vi "Thorlabs_TDC001.findReference.vi"(0 "i ref in":refnum<vi>, 5 "error in (no error)":errorcluster) -> (14 "i ref out":refnum<vi>, 19 "error out":errorcluster)   [LabVIEW 2014, in "Thorlabs_TDC001.lvlib"]
doc: "This is the constructor of a class.\n\nLicense Agreement for this software:\n\nCopyright (C)\nGesellschaft für Schwerionenforschung, GSI\nPlanckstr. 1\n64291 Darmstadt\nGermany\n\nContact: D.Beck@gsi.de \n\nThis program is free software; you can redistribute it and/or modify it under the terms of the \nGNU General Public License as published by the Free Software Foundation; either version 2 of \nthe license, or (at your option) any later version.\n\nThis program is distributed in the hope that it will be useful, but WITHOUT ANY WARRANTY; \nwithout even the implied warranty of MERCHANTABILITY or FITNESS FOR A PARTICULAR PURPOSE. See the GNU General License for more details (http://www.gnu.org).\n\nGesellschaft für Schwerionenforschung, GSI\nPlanckstr. 1, 64291 Darmstadt, Germany\nFor all questions and ideas contact: M.Richter@gsi.de, H.Brand@gsi.de or D.Beck@gsi.de.\nLast update: 16-JUN-2004"
uses:
  Thorlabs_TDC001.lvlib
panel:
  in  "MG17Motor":refnum<k7>(container)
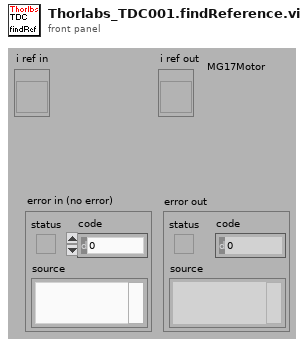
[diagram p1: front panel]
types:
  T1 = typedef "Thorlabs_TDC001.lvlib/Thorlabs_TDC001.i attribute.ctl" = cluster{"SerialNo":i32, "ChannelID":i32}
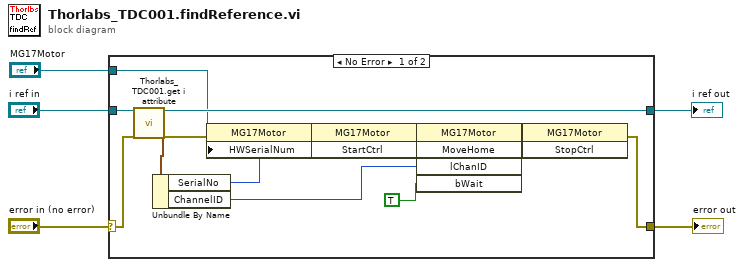
[diagram p0: block diagram]
diagram:
  n1 = case shown="No Error" "error in (no error)" {
    selector: "error in (no error)" -> [w20 w23]
    tunnel: [w6 w23] -> w5
    tunnel: "i ref in" -> [w21 w22]
    tunnel: [w19 w22] -> w2
    tunnel: "MG17Motor" -> [w16 _]
    frame No Error {
      n2 = call "Thorlabs_TDC001.get i attribute.vi"("i ref in"=w21, "error in (no error)"=w20) -> ("i ref out"=w19:refnum<vi>, "i attribute"=w18:T1, "error out"=w15:errorcluster)  [unwired: 15 in]
      n3 = Unbundle By Name(w18) -> ("SerialNo"=w14:i32, "ChannelID"=w9:i32)
      n4 = property class="MG17Motor"(reference=w16, error in=w15, "HWSerialNum"=w14) -> (reference out=w13:refnum<k7>, error out=w12:errorcluster)
      n5 = invoke class="MG17Motor" method="StartCtrl"(reference=w13, error in=w12) -> (reference out=w11:refnum<k7>, error out=w10:errorcluster)  [unwired: 1 in, 1 out]
      n6 = invoke class="MG17Motor" method="MoveHome"(reference=w11, error in=w10, "lChanID"=w9, "bWait"=TRUE) -> (reference out=w8:refnum<k7>, error out=w7:errorcluster)  [unwired: 1 in, 3 out]
      n7 = invoke class="MG17Motor" method="StopCtrl"(reference=w8, error in=w7) -> (error out=w6:errorcluster)  [unwired: 1 in, 2 out]
    }
    frame Error {
    }
  }
  "error out" <- w5
  "i ref out" <- w2
